vi "Get Nested Global Log Instance.vi"(8 "error in (no error)":errorcluster) -> (0 "error out":errorcluster, 3 "Nested Global Log Instance Reference":refnum<class "LoggerReference.lvclass">)   [LabVIEW 2020, in "Singleton Event Log.lvlib"]
doc: "Obtain a nested instance of the global log. Log events passed to this instance will be propagated to the global log instance, however as this is a nested instance, closing this instance will not close the global log. Similarly, any sinks added to this instance will capture events specific to this instance only."
uses:
  <vilib>/gpm_packages/@cs/event-logger/Source/Composed Log/Singleton Event Log/Singleton Event Log.lvlib
  <vilib>/gpm_packages/@cs/event-logger/Source/Composed Log/LoggerReference/LoggerReference.lvclass
  <vilib>/gpm_packages/@cs/event-logger/Source/Composed Log/LoggerReference/LoggerReference.lvclass/LoggerReference.ctl
  b2f05d58-65df-4e80-8f90-78513ac31376.vi
  <vilib>/gpm_packages/@cs/event-logger/Source/Composed Log/LoggerReference/Return Aggregate Queues.vi
  <vilib>/gpm_packages/@cs/event-logger/Source/Composed Log/LoggerReference/Add Aggregate Log.vi
  b2f05d58-65df-4e80-8f90-78513ac31376.vi/2eb4f93f-93a6-47e8-8693-c1e51e99c0d7.vi
  <vilib>/gpm_packages/@cs/event-logger/Source/Composed Log/LoggerReference/Send Add Sink.vi
  <vilib>/gpm_packages/@cs/event-logger/Source/Composed Log/Application Logger/Launch Worker Loop.vi
  <vilib>/gpm_packages/@cs/event-logger/Source/Composed Log/LoggerReference/Initialize Logger Instance.vi
  <vilib>/gpm_packages/@cs/event-logger/Source/Composed Log/Log Sink/Log Sink.lvclass
  <vilib>/gpm_packages/@cs/event-logger/Source/Composed Log/IErrorFormat/IErrorFormat.lvclass
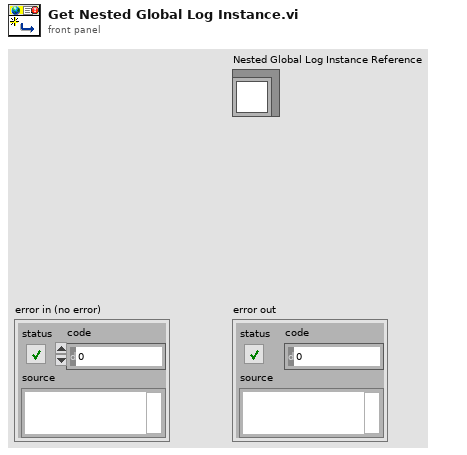
[diagram p1: front panel]
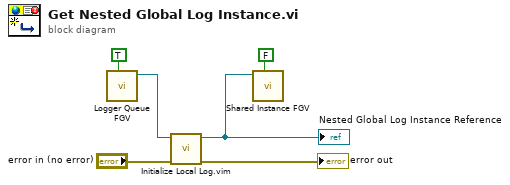
[diagram p0: block diagram]
diagram:
  n1 = call <vilib>:"Logger Queue FGV.vi"("Read?"=TRUE) -> ("LogReference Instance Out"=w5:refnum<class "LoggerReference.lvclass">)  [unwired: 10 in]
  n2 = call "Initialize Local Log.vim"("error in (no error)"="error in (no error)", "Parent Log Reference"=w5) -> ("error out"=→"error out":errorcluster, "Log Instance Reference"=w4:refnum<class "LoggerReference.lvclass">)  [unwired: 7 in, 1 out]
  "Nested Global Log Instance Reference" <- w4
  n3 = call <vilib>:"Shared Instance FGV.vi"("Read?"=FALSE, "LogReference Instance"=w4) -> ()  [unwired: 9 in, 1 out]
